vi "LeCroyAVG_Arm.vi"(7 "EXT AVG":bool, 8 "error in":errorcluster, 10 "Avg Num":i32=1, 11 "LeCroy":refnum<visa-resource-name>) -> (0 "error out":errorcluster, 3 "LeCroy":refnum<visa-resource-name>)   [LabVIEW 2022 SP3]
uses:
  <instrlib>/LeCroy Wave Series/LeCroy Wave Series.lvlib
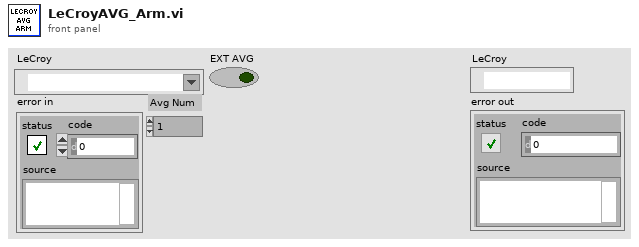
[diagram p1: front panel]
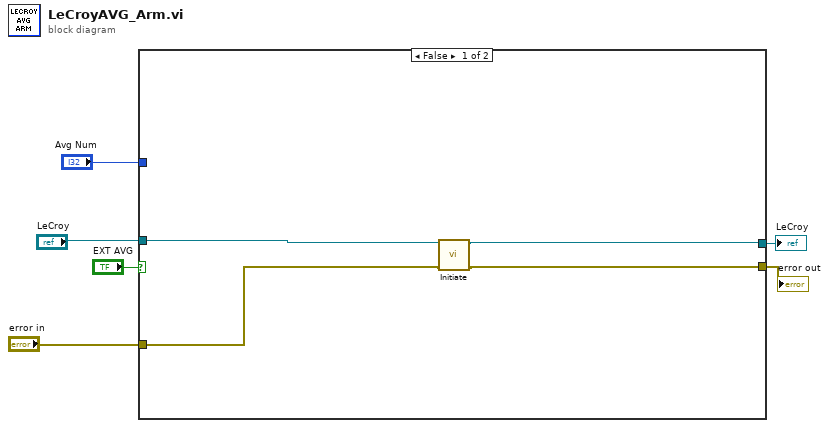
[diagram p0: block diagram]
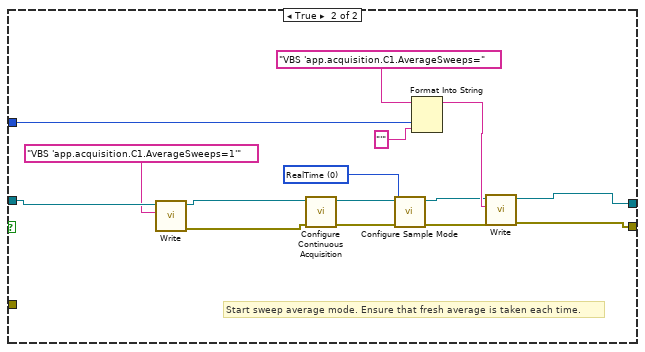
[diagram p2: hidden frame]
diagram:
  n1 = case shown="False" "EXT AVG" {
    tunnel: "LeCroy" -> [w10 w18]
    tunnel: "error in" -> [w7 _]
    tunnel: "Avg Num" -> [_ w22]
    tunnel: [w9 w14] -> w3
    tunnel: [w8 w13] -> w2
    frame False {
      n2 = call <instrlib>:"Initiate.vi"("error in (no error)"=w7, "VISA resource name"=w10) -> ("error out"=w8:errorcluster, "VISA resource name out"=w9:refnum<visa-resource-name>)  [unwired: 8 in]
    }
    frame True {
      w23 = u16 0 items=["RealTime", "RIS", "Sequence", "Roll", "WaveStream"] ("Sample Mode (0: RealTime)")
      # "Start sweep average mode. Ensure that fresh average is taken each time."
      n3 = call <instrlib>:"Write.vi"("Write Buffer"="VBS 'app.acquisition.C1.AverageSweeps=1'", "VISA resource name"=w18) -> ("error out"=w16:errorcluster, "VISA resource name out"=w17:refnum<visa-resource-name>)  [unwired: 7 in, 1 out]
      n4 = call <instrlib>:"Configure Continuous Acquisition.vi"("error in (no error)"=w16, "VISA resource name"=w17) -> ("error out"=w25:errorcluster, "VISA resource name out"=w24:refnum<visa-resource-name>)  [unwired: 8 in]
      n5 = call <instrlib>:"Configure Sample Mode.vi"("error in (no error)"=w25, "Sample Mode (0: RealTime)"=w23, "VISA resource name"=w24) -> ("error out"=w19:errorcluster, "VISA resource name out"=w20:refnum<visa-resource-name>)  [unwired: 7 in]
      n6 = Format Into String(initial string="VBS 'app.acquisition.C1.AverageSweeps=", w22, "'") -> (resulting string=w21:string)  [unwired: 2 in, 1 out]
      n7 = call <instrlib>:"Write.vi"("error in (no error)"=w19, "Write Buffer"=w21, "VISA resource name"=w20) -> ("error out"=w13:errorcluster, "VISA resource name out"=w14:refnum<visa-resource-name>)  [unwired: 6 in, 1 out]
    }
  }
  "LeCroy" <- w3
  "error out" <- w2
